vi "3_AdvancedDemo_MHT3.vi"() -> ()   [LabVIEW 2010]
uses:
  Types/MH_UIThread_Cmds.ctl
  _lib/PQ/MultiHarp/MH_InitInfo.ctl
  Types/MH_UIThread_Data.ctl
  Types/MH_InputChannel.ctl
  _lib/PQ/MultiHarp/MH_RefSource.ctl
  _lib/PQ/MultiHarp/mhlib_x86_x64_UIThread.llb/MH_DllPath_global.vi
  <vilib>/Utility/error.llb/DialogType.ctl
  Types/MH_DataProcThread_QCmds.ctl
  Types/MH_DataProcThread_QData.ctl
  Types/MH_VisThread_QCmds.ctl
  Types/MH_VisThread_QData.ctl
  Types/MH_VisThread_Data.ctl
  _lib/PQ/MultiHarp/MH_LibVersion_global.vi
  _lib/PQ/MultiHarp/MH_MeasMode.ctl
panel:
  in  "Settings":bool=TRUE
  in  "Run continuously":bool caption="Conti."
  in  "Start":bool
  in  "Scale":bool
  out "CountRates":i32[](graph)
  in  "HistoAcqTime":dbl=1.0 caption="Int.Time    s" min=0.1 max=360000.0 step=0.1
  in  "AcqTime":i32=360000000 caption="T3Acq.   ms" min=1 max=360000 step=1
  in  "Binning":i32(ring) caption="Resol.      ps" items=["80", "160", "320", "640", "1280", "2560", "5120", "10240", "20480", "40960", "81920", "163840", "327680", "655360", "1310720", "2621440", "5242880", "10485760", "20971520", "41943040", "83886080", "167772160", "335544320", "671088640", "1342177280", "2684354560"]
  in  "HistoOffset":i32 caption="Offset      ns" min=0 max=100000000 step=1
  out "DeltaT":dbl=3.2767475720388473 caption="Resol.     ms" format="%.2f"
  in  "BitShift":i32=15 min=0 max=32 step=1
  in  "OvlLevel":i32=65536 caption="Ovl.Level" min=1024 max=65536 step=1024
  in  "StopOvl.":bool=TRUE
  out "TTraceGraph":T1(graph)={0.0, "Resolution"=0.0032767475720388473, "Histogram"=[]}
  out "HistoGraph":cluster{dbl, "Resol":dbl, "Histos":u32[][]}(graph)={0.0, "Resol"=0.08, "Histos"=[]}
  in  "SyncEdge":i32(ring) caption="Edge" items=["falling", "rising"]
  in  "SyncDivider":i32(ring)=3 caption="Divider" items=["1", "2", "4", "8", "16"]
  in  "SyncOffset":i32 caption="Offset      ps" min=-99999 max=99999 step=1
  in  "SyncLevel":i32=-50 caption="Level      mV" min=-1200 max=1200 step=1
  in  "Channels":T2[](array[typedef])=[{"Name"="Inp.Chan 1", "Enable"=TRUE, "Offset"=0, "Level"=-50, "Edge"=0}, {"Name"="Inp.Chan 2", "Enable"=TRUE, "Offset"=0, "Level"=-50, "Edge"=0}, {"Name"="Inp.Chan 3", "Enable"=TRUE, "Offset"=0, "Level"=-50, "Edge"=0}, {"Name"="Inp.Chan 4", "Enable"=TRUE, "Offset"=0, "Level"=-50, "Edge"=0}, {"Name"="Inp.Chan 5", "Enable"=TRUE, "Offset"=0, "Level"=-50, "Edge"=0}, {"Name"="Inp.Chan 6", "Enable"=TRUE, "Offset"=0, "Level"=-50, "Edge"=0}, {"Name"="Inp.Chan 7", "Enable"=TRUE, "Offset"=0, "Level"=-50, "Edge"=0}, {"Name"="Inp.Chan 8", "Enable"=TRUE, "Offset"=0, "Level"=-50, "Edge"=0}] {"Edge" items=["falling", "rising"]; "Offset" min=-99999 max=99999 step=80; "Level" min=-1200 max=1200 step=1}
  out "SyncRate":string="Sync Rate: 10000160 cps\n"
  out "OverRun":bool caption="Overrun:"
  out "Status":string="Elements in Q: 0"
  # "Histogram"
  # "Time Trace"
  # "Sync"
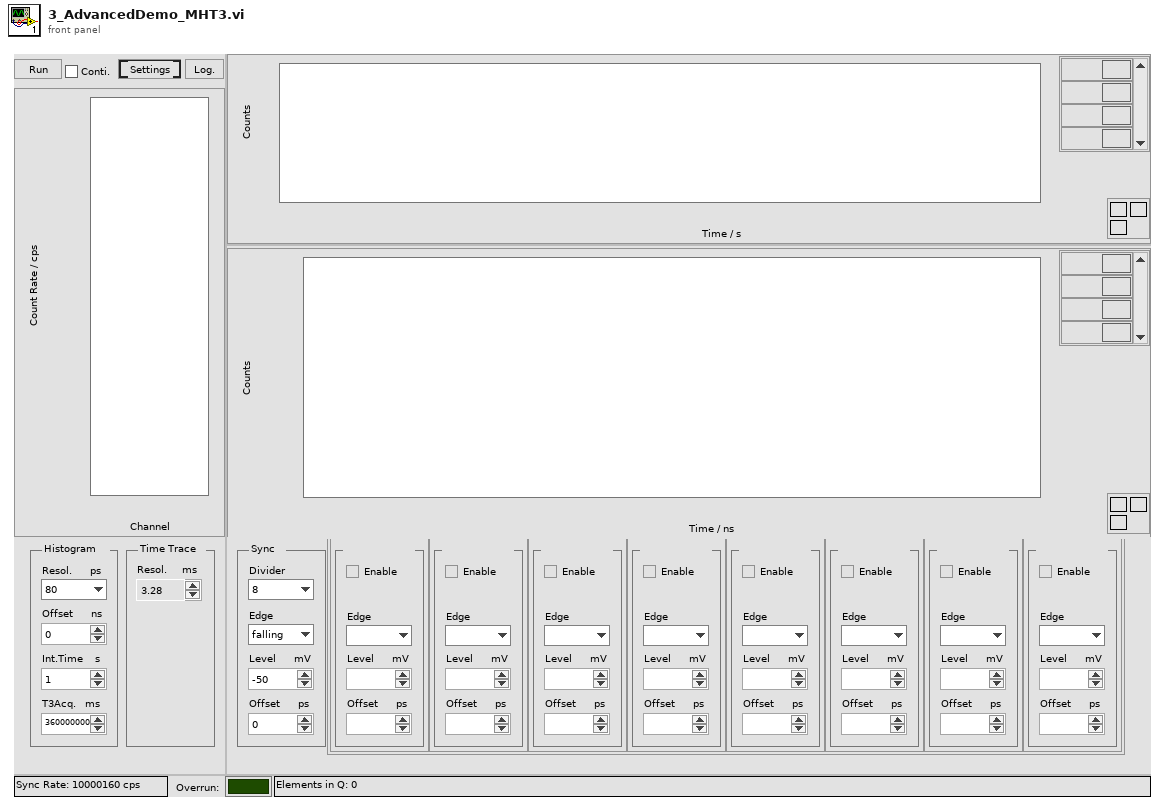
[diagram p1: front panel]
types:
  T1 = cluster{dbl, "Resolution":dbl, "Histogram":u32[][]}
  T2 = typedef "MH_InputChannel.ctl" = cluster{"Name":string, "Enable":bool, "Offset":i32, "Level":i32, "Edge":i32}
  T3 = typedef "MH_DataProcThread_QCmds.ctl" = enum16{"Exit", "Proc", "Init", "SetShift", "SetNumChannels", "SetHistAcqTime"}
  T4 = typedef "MH_VisThread_Data.ctl" = cluster{"Resol":dbl, "DeltaT":dbl, "NumChannels":i32}
  T5 = typedef "MH_VisThread_QData.ctl" = cluster{"Histos":u32[][], "Cmd":T6, "TimeTrace":u32[][], "Bin":i32, "Total bin":u64, "Status":string, "Resol":dbl, "DeltaT":dbl, "nChannels":i32}
  T6 = typedef "MH_VisThread_QCmds.ctl" = enum16{"_none_", "Resol", "nChannels", "DeltaT", "Histo", "TTrace", "Status"}
  T7 = typedef "MH_DataProcThread_QData.ctl" = cluster{"Cmd":T3, "nActual":i32, "Buffer":u32[], "TickCount":u32, "Param":i32}
  T8 = typedef "MH_UIThread_Data.ctl" = cluster{"Init Info":T9, "DevIdx":i32, "SyncDivider":i32, "SyncOffset":i32, "SyncLevel":i32, "Channels":T2[], "CurrentChannels":i32[], "AcqTime":i32, "Binning":i32, "HistoOffset":i32, "HistoLen":i32, "StopOvl.":bool, "OvlLevel":u32, "SyncEdge":i32, "StartMeas":bool, "HistoLength":i32, "Resolution":dbl, "Run cont.":bool, "Status":string, "SyncRate":i32, "BitShift":i32, "HistoAcqTime":dbl}
  T9 = typedef "MH_InitInfo.ctl" = cluster{"Library Version":string, "Serial No.":string, "Model":string, "Partnum":string, "Version":string, "features":i32, "nchannels":i32, "Base Resolution":dbl, "Bin Steps":i32}
  T10 = typedef "MH_UIThread_Cmds.ctl" = enum16{"Idle", "Init", "SetInpChanEnable", "SetInpChanOffset", "SetInpChanTrg", "SetSyncDivider", "SetSyncTrg", "SetSyncOffset", "SetBinning", "SetHistoOffset", "SetHistoLen", "SetStopOvl", "SetBitShift", "SetHistoAcqTime", "GetRates", "GetAllRates", "StartMeas", "StopMeas", "AbortMeas", "GetResolution", "GetHistos", "GetAllHistos", "ReadFiFo", "WriteStatus", "Resize", "EnableControls", "DisableControls", "Error", "Exit"}
  T11 = enum8{"Enabled", "Disabled", "Disabled and Grayed Out"}
  T12 = typedef "MH_MeasMode.ctl" = i32
  T13 = typedef "MH_RefSource.ctl" = enum16{"INTERNAL", "EXTERNAL_10MHZ", "WR_MASTER_GENERIC", "WR_SLAVE_GENERIC", "WR_GRANDM_GENERIC", "EXTN_GPS_PPS", "EXTN_GPS_PPS_UART", "WR_MASTER_MHARP", "WR_SLAVE_MHARP", "WR_GRANDM_MHARP"}
  T14 = typedef "DialogType.ctl" = u16
  T15 = cluster{"T0":dbl, "dt":dbl, "TimeTrace_out":u32[][]}
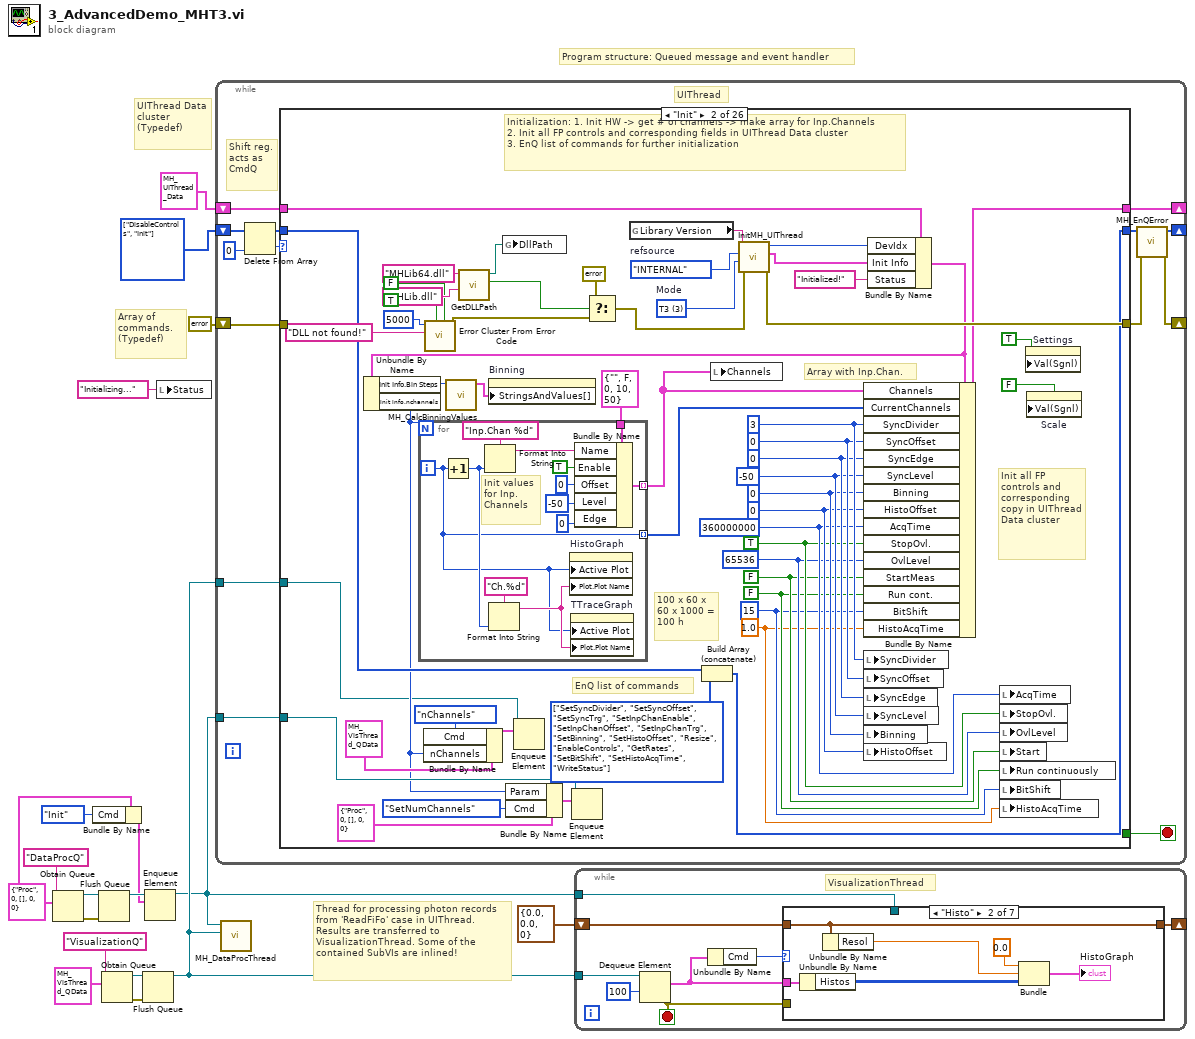
[diagram p0: block diagram]
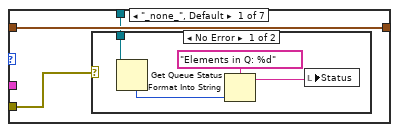
[diagram p2: hidden frame]
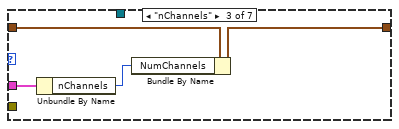
[diagram p4: hidden frame]
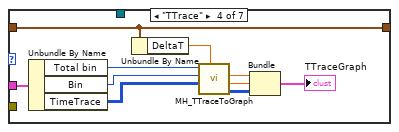
[diagram p5: hidden frame]
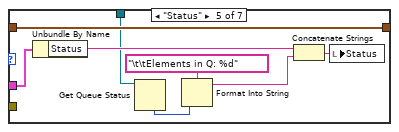
[diagram p6: hidden frame]
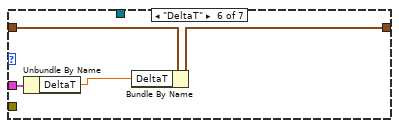
[diagram p7: hidden frame]
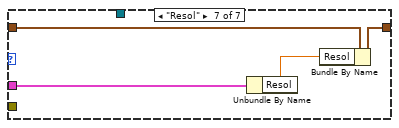
[diagram p8: hidden frame]
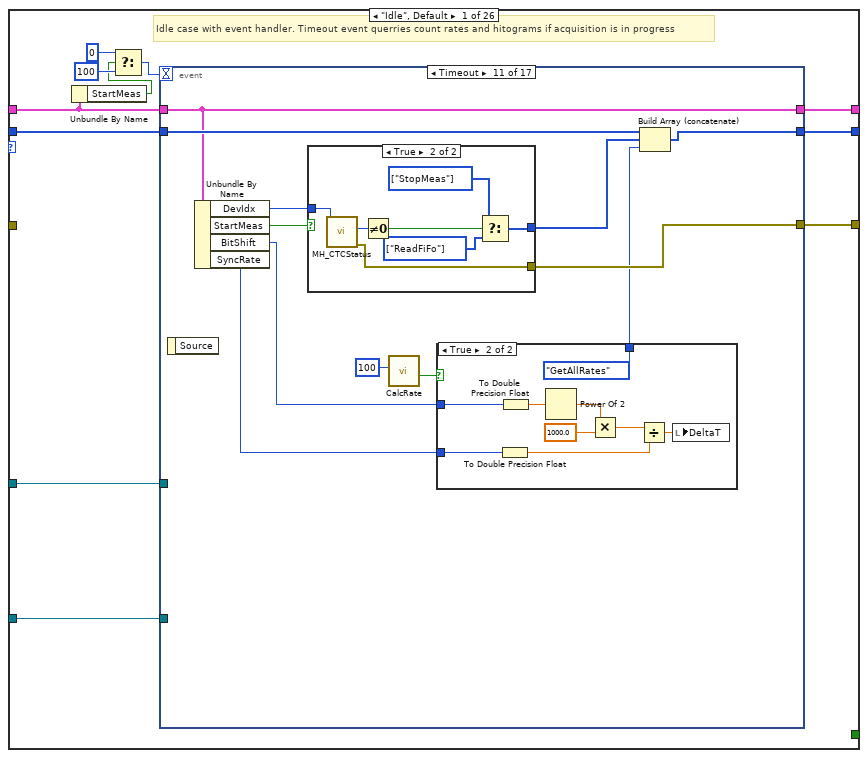
[diagram p9: hidden frame]
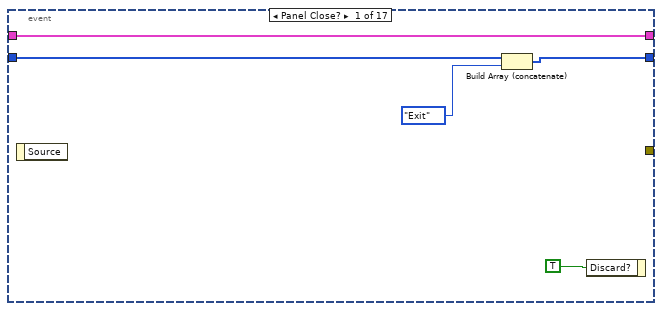
[diagram p10: hidden frame]
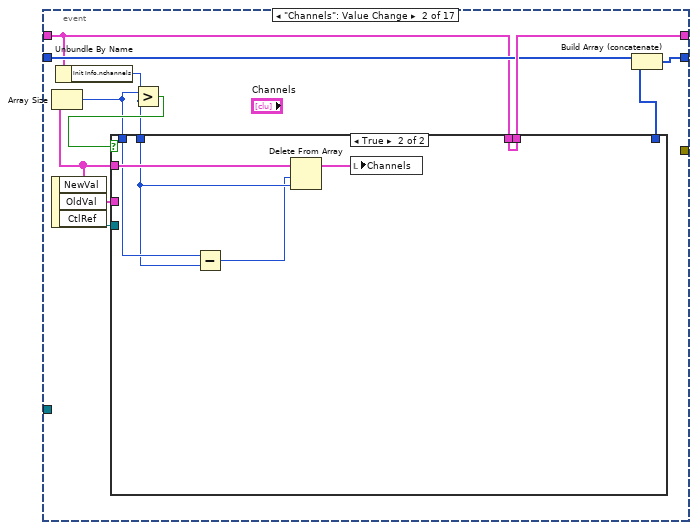
[diagram p11: hidden frame]
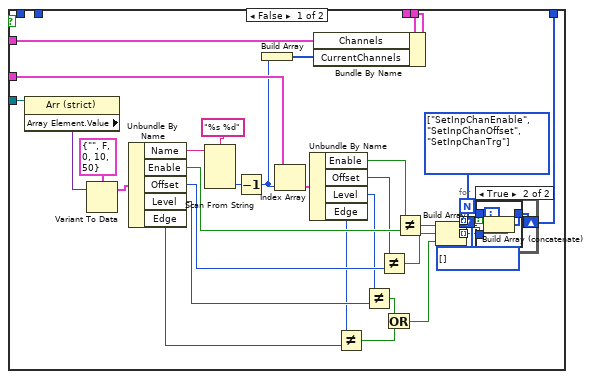
[diagram p12: hidden frame]
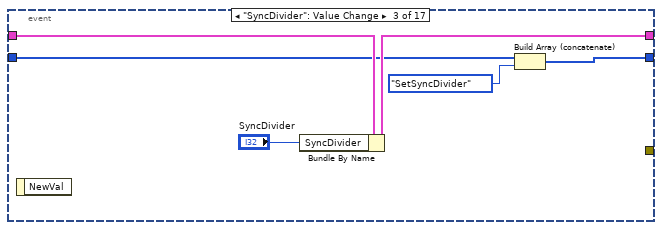
[diagram p14: hidden frame]
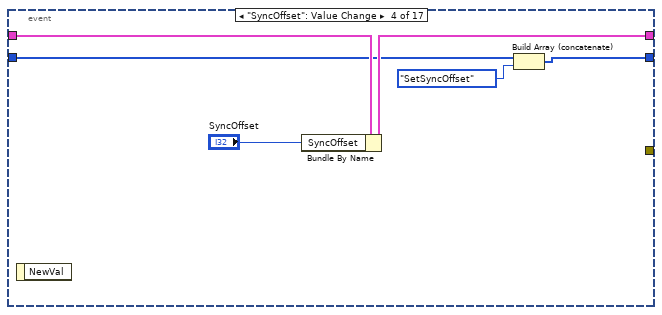
[diagram p15: hidden frame]
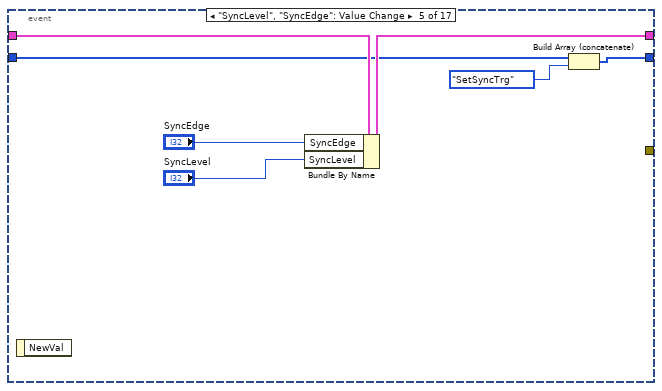
[diagram p16: hidden frame]
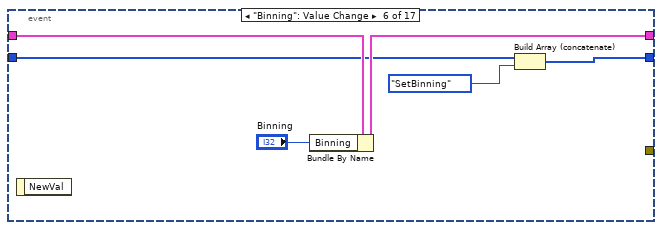
[diagram p17: hidden frame]
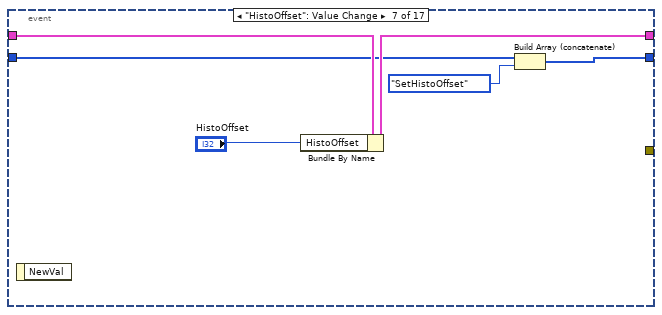
[diagram p18: hidden frame]
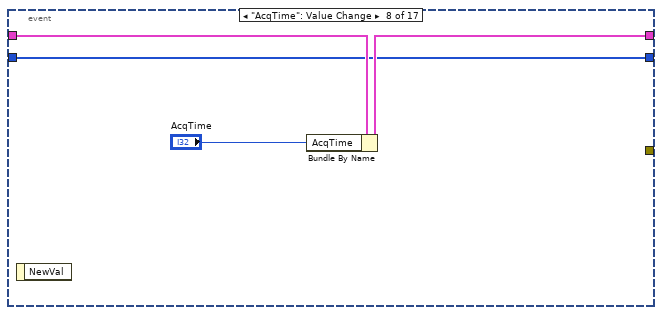
[diagram p19: hidden frame]
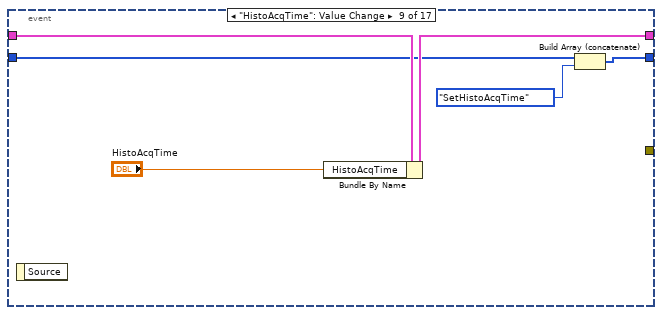
[diagram p20: hidden frame]
diagram:
  w4 = T7 {"Cmd"=enum."Proc", "nActual"=0, "Buffer"=[], "TickCount"=0, "Param"=0} ("MH_DataProcThread_QData")
  w17 = T10[] [enum."DisableControls", enum."Init"] items=["Idle", "Init", "SetInpChanEnable", "SetInpChanOffset", "SetInpChanTrg", "SetSyncDivider", "SetSyncTrg", "SetSyncOffset", "SetBinning", "SetHistoOffset", "SetHistoLen", "SetStopOvl", "SetBitShift", "SetHistoAcqTime", "GetRates", "GetAllRates", "StartMeas", "StopMeas", "AbortMeas", "GetResolution", "GetHistos", "GetAllHistos", "ReadFiFo", "WriteStatus", "Resize", "EnableControls", "DisableControls", "Error", "Exit"]
  # "Thread for processing photon records from 'ReadFiFo' case in UIThread. Results are transferred to VisualizationThread. Some of the contained SubVIs are inlined!"
  # "Array of commands.\n(Typedef)"
  # "Program structure: Queued message and event handler"
  # "UIThread Data cluster\n(Typedef)"
  n1 = Obtain Queue(name (unnamed)="DataProcQ", element data type=w4) -> (queue out=w14:refnum<queue>, error out=w13:errorcluster)  [unwired: 3 in, 1 out]
  n2 = Bundle By Name(cluster=w4, "Cmd"=MH_DataProcThread_QCmds."Init") -> (w2:T7)
  n3 = Flush Queue(queue=w14, error in (no error)=w13) -> (queue out=w5:refnum<queue>)  [unwired: 2 out]
  n4 = Obtain Queue(name (unnamed)="VisualizationQ", element data type=T5 {"Histos"=[], "Cmd"=enum."_none_", "TimeTrace"=[], "Bin"=0, "Total bin"=0, "Status"="", "Resol"=0.0, "DeltaT"=0.0, "nChannels"=0} ("MH_GUIThread_QData")) -> (queue out=w12:refnum<queue>, error out=w11:errorcluster)  [unwired: 3 in, 1 out]
  n5 = Flush Queue(queue=w12, error in (no error)=w11) -> (queue out=w7:refnum<queue>)  [unwired: 2 out]
  n6 = Enqueue Element(queue=w5, element=w2) -> (queue out=w1:refnum<queue>)  [unwired: 2 in, 2 out]
  n7 = local write "Status"("Initializing..." ("Status")) -> ()
  n8 = while {
    shift-right: [w21] -> _
    shift-left: w17 -> [w28]
    shift-right: [w31] -> _
    shift-left: T8 {"Init Info"={"Library Version"="", "Serial No."="", "Model"="", "Partnum"="", "Version"="", "features"=0, "nchannels"=0, "Base Resolution"=0.0, "Bin Steps"=0}, "DevIdx"=0, "SyncDivider"=1, "SyncOffset"=0, "SyncLevel"=50, "Channels"=[], "CurrentChannels"=[], "AcqTime"=1, "Binning"=1, "HistoOffset"=1, "HistoLen"=1024, "StopOvl."=FALSE, "OvlLevel"=1024, "SyncEdge"=10, "StartMeas"=FALSE, "HistoLength"=0, "Resolution"=0.0, "Run cont."=FALSE, "Status"="", "SyncRate"=0, "BitShift"=0, "HistoAcqTime"=0.0} -> [w30]
    shift-right: [w23] -> _
    shift-left: errorcluster {"status"=FALSE, "code"=0, "source"=""} ("error IO") -> [w29]
    tunnel: w1 -> [w20]
    tunnel: w7 -> [w19]
    stop <- w32 stop-if-true
    # "Shift reg.\nacts as\nCmdQ"
    # "UIThread"
    n9 = Delete From Array(array=w28, index=0) -> (deleted portion=w26:T10, array with subset deleted=w25:T10[])  [unwired: 1 in]
    n10 = case shown="\"Init\"" w26 {
      tunnel: [w43 w283 w307 w321 w335 w352 w361 w363 w370 w378 w385 w405 w417 w427 w439 w459 w465 w478 w495 w496 w522 w535 w542 w554 w560 w566] -> w22
      tunnel: [_ _ _ _ _ _ _ _ _ _ _ _ _ _ _ _ _ _ _ _ _ _ _ _ _ TRUE] -> w32
      tunnel: [w42 w264 w310 w324 w338 w354 w362 w367 w374 w379 w386 w390 w407 w421 w431 w463 w468 w480 w491 w506 w521 w523 w541 w553 w561 w569] -> w31
      tunnel: w30 -> [w39 w269 w310 w324 w338 w354 w362 w367 w374 w379 w386 w390 w407 w421 w432 w463 w469 w481 w492 w506 w521 w523 w541 w553 w561 w569]
      tunnel: [w40 w288 w308 w322 w336 w350 w360 w366 w373 w377 w384 _ _ w420 w438 w462 w471 w483 w493 w501 _ _ _ _ _ w567] -> w24
      tunnel: w29 -> [_ _ _ _ _ _ _ _ _ _ _ _ _ _ _ _ _ _ _ _ _ _ _ _ w562 _]
      tunnel: w25 -> [w41 w285 w307 w321 w335 w352 w361 w363 w369 w378 w385 w405 w417 w427 w439 w460 w466 w478 w495 w497 w522 w535 w542 w554 _ w566]
      tunnel: w20 -> [w34 w262 _ _ _ _ _ _ _ _ _ w391 w408 _ _ w456 _ _ _ w498 _ _ _ _ _ w565]
      tunnel: w19 -> [w33 w254 _ _ _ _ _ _ _ _ _ w392 _ _ _ _ _ _ w488 _ _ _ _ _ _ w564]
      frame "Idle", Default {
        # "Idle case with event handler. Timeout event querries count rates and hitograms if acquisition is in progress"
        n11 = Unbundle By Name(w39) -> ("StartMeas"=w37:bool)
        n12 = Select(t=0, s=w37, f=100) -> (s? t:f=w36:i32)
        n13 = event shown="[10] Timeout" {
          selector: _ -> [_ _ _ _ _ _ _ _ _ _ _ _ _ _ _ _ _]
          dyn-events: _ -> [_ _ _ _ _ _ _ _ _ _ _ _ _ _ _ _ _]
          timeout: w36 -> [_ _ _ _ _ _ _ _ _ _ _ _ _ _ _ _ _]
          tunnel: [w44 w54 w105 w111 w118 w125 w131 w136 w141 w148 w163 w181 w193 w211 w217 w225 w235] -> w43
          tunnel: [w47 w57 w109 w115 w122 w128 w134 w138 w144 w151 w162 w185 w192 w209 w216 w224 w238] -> w42
          tunnel: w39 -> [w47 w53 w110 w116 w123 w129 w135 w139 w145 w152 w162 w186 w190 w210 w216 w224 w238]
          tunnel: w41 -> [w46 w56 w107 w113 w120 w127 w133 w136 w142 w150 w164 w182 w194 w211 w217 w225 w236]
          tunnel: [_ _ _ _ _ _ _ _ _ _ w158 _ _ _ _ _ _] -> w40
          tunnel: w34 -> [_ _ _ _ _ _ _ _ _ _ _ _ _ _ _ _ _]
          tunnel: w33 -> [_ _ _ _ _ _ _ _ _ _ _ _ _ _ _ _ _]
          event Panel Close? {
            n14 = event-data() -> ()  [unwired: 1 in, 1 out]
            n15 = Build Array (concatenate)(w46, MH_UIThread_Cmds."Exit") -> (w44:T10[])
            n16 = event-data("Discard?"=TRUE) -> ()  [unwired: 1 in, 1 out]
          }
          event "Channels": Value Change {
            n17 = event-data() -> ("NewVal"=w52:T2[], "OldVal"=w58:T2[], "CtlRef"=w59:refnum<vi>)  [unwired: 1 in]
            n18 = Array Size(array=w52) -> (size(s)=w49:i32)
            n19 = Unbundle By Name(w53) -> ("Init Info.nchannels"=w50:i32)
            n20 = Greater?(x=w49, y=w50) -> (0:w51:bool)
            n21 = case shown="True" w51 {
              tunnel: w59 -> [w90 _]
              tunnel: w58 -> [w84 _]
              tunnel: [w67 w104] -> w57
              tunnel: [w65 _] -> w55
              tunnel: w53 -> [w62 w104]
              tunnel: w52 -> [w61 w103]
              tunnel: w50 -> [_ w101]
              tunnel: w49 -> [_ w102]
              frame False {
                w60 = T10[] [] items=["Idle", "Init", "SetInpChanEnable", "SetInpChanOffset", "SetInpChanTrg", "SetSyncDivider", "SetSyncTrg", "SetSyncOffset", "SetBinning", "SetHistoOffset", "SetHistoLen", "SetStopOvl", "SetBitShift", "SetHistoAcqTime", "GetRates", "GetAllRates", "StartMeas", "StopMeas", "AbortMeas", "GetResolution", "GetHistos", "GetAllHistos", "ReadFiFo", "WriteStatus", "Resize", "EnableControls", "DisableControls", "Error", "Exit"] ("Array")
                w68 = T10[] [enum."SetInpChanEnable", enum."SetInpChanOffset", enum."SetInpChanTrg"] items=["Idle", "Init", "SetInpChanEnable", "SetInpChanOffset", "SetInpChanTrg", "SetSyncDivider", "SetSyncTrg", "SetSyncOffset", "SetBinning", "SetHistoOffset", "SetHistoLen", "SetStopOvl", "SetBitShift", "SetHistoAcqTime", "GetRates", "GetAllRates", "StartMeas", "StopMeas", "AbortMeas", "GetResolution", "GetHistos", "GetAllHistos", "ReadFiFo", "WriteStatus", "Resize", "EnableControls", "DisableControls", "Error", "Exit"]
                n22 = property class="Arr (strict)"(reference=w90) -> ("Array Element.Value"=w89:variant)  [unwired: 1 in, 2 out]
                n23 = Variant To Data(Variant=w89, type=T2 {"Name"="", "Enable"=FALSE, "Offset"=0, "Level"=10, "Edge"=50} ("Channel")) -> (data=w66:cluster{})  [unwired: 1 in, 1 out]
                n24 = Unbundle By Name(w66) -> ("Name"=w87:string, "Enable"=w81:bool, "Offset"=w79:i32, "Level"=w77:i32, "Edge"=w75:i32)
                n25 = Scan From String(format string="%s %d", input string=w87) -> (output 2=w85:i32)  [unwired: 5 in, 3 out]
                n26 = Decrement(x=w85) -> (x-1=w64:i32)
                n27 = Build Array(w64) -> (w63:i32[])
                n28 = Index Array(array=w84, index=w64) -> (element=w83:T2)
                n29 = Unbundle By Name(w83) -> ("Enable"=w82:bool, "Offset"=w80:i32, "Level"=w78:i32, "Edge"=w76:i32)
                n30 = Bundle By Name(cluster=w62, "Channels"=w61, "CurrentChannels"=w63) -> (w67:T8)
                n31 = Not Equal?(x=w76, y=w75) -> (x != y?=w70:bool)
                n32 = Not Equal?(x=w78, y=w77) -> (x != y?=w71:bool)
                n33 = Not Equal?(x=w80, y=w79) -> (x != y?=w73:bool)
                n34 = Or(x=w71, y=w70) -> (x .or. y?=w69:bool)
                n35 = Not Equal?(x=w82, y=w81) -> (x != y?=w74:bool)
                n36 = Build Array(w74, w73, w69) -> (w72:bool[])
                n37 = for {
                  tunnel: w72 -> [w93] mode=indexing
                  tunnel: w68 -> [w94] mode=indexing
                  shift-right: [w91] -> w65
                  shift-left: w60 -> [w92]
                  n38 = case shown="True" w93 {
                    tunnel: w92 -> [w95 w97]
                    tunnel: w94 -> [_ w96]
                    tunnel: [w95 w98] -> w91
                    frame False {
                    }
                    frame True {
                      n39 = Build Array (concatenate)(w97, w96) -> (w98:T10[])
                    }
                  }
                }
              }
              frame True {
                n40 = Subtract(x=w102, y=w101) -> (x-y=w100:i32)
                n41 = Delete From Array(array=w103, length=w100, index=w101) -> (array with subset deleted=w99:T2[])  [unwired: 1 out]
                n42 = local write "Channels"(w99) -> ()
              }
            }
            n43 = Build Array (concatenate)(w56, w55) -> (w54:T10[])
          }
          event "SyncDivider": Value Change {
            n44 = event-data() -> ()  [unwired: 1 in, 1 out]
            n45 = Bundle By Name(cluster=w110, "SyncDivider"="SyncDivider") -> (w109:T8)
            n46 = Build Array (concatenate)(w107, MH_UIThread_Cmds."SetSyncDivider") -> (w105:T10[])
          }
          event "SyncOffset": Value Change {
            n47 = event-data() -> ()  [unwired: 1 in, 1 out]
            n48 = Bundle By Name(cluster=w116, "SyncOffset"="SyncOffset") -> (w115:T8)
            n49 = Build Array (concatenate)(w113, MH_UIThread_Cmds."SetSyncOffset") -> (w111:T10[])
          }
          event "SyncLevel", "SyncEdge": Value Change {
            n50 = event-data() -> ()  [unwired: 1 in, 1 out]
            n51 = Bundle By Name(cluster=w123, "SyncEdge"="SyncEdge", "SyncLevel"="SyncLevel") -> (w122:T8)
            n52 = Build Array (concatenate)(w120, MH_UIThread_Cmds."SetSyncTrg") -> (w118:T10[])
          }
          event "Binning": Value Change {
            n53 = event-data() -> ()  [unwired: 1 in, 1 out]
            n54 = Bundle By Name(cluster=w129, "Binning"="Binning") -> (w128:T8)
            n55 = Build Array (concatenate)(w127, MH_UIThread_Cmds."SetBinning") -> (w125:T10[])
          }
          event "HistoOffset": Value Change {
            n56 = event-data() -> ()  [unwired: 1 in, 1 out]
            n57 = Bundle By Name(cluster=w135, "HistoOffset"="HistoOffset") -> (w134:T8)
            n58 = Build Array (concatenate)(w133, MH_UIThread_Cmds."SetHistoOffset") -> (w131:T10[])
          }
          event "AcqTime": Value Change {
            n59 = event-data() -> ()  [unwired: 1 in, 1 out]
            n60 = Bundle By Name(cluster=w139, "AcqTime"="AcqTime") -> (w138:T8)
          }
          event "HistoAcqTime": Value Change {
            n61 = event-data() -> ()  [unwired: 1 in, 1 out]
            n62 = Bundle By Name(cluster=w145, "HistoAcqTime"="HistoAcqTime") -> (w144:T8)
            n63 = Build Array (concatenate)(w142, MH_UIThread_Cmds."SetHistoAcqTime") -> (w141:T10[])
          }
          event "OvlLevel", "StopOvl.": Value Change {
            n64 = event-data() -> ()  [unwired: 1 in, 1 out]
            n65 = Bundle By Name(cluster=w152, "StopOvl."="StopOvl.", "OvlLevel"="OvlLevel") -> (w151:T8)
            n66 = Build Array (concatenate)(w150, MH_UIThread_Cmds."SetStopOvl") -> (w148:T10[])
          }
          event Timeout {
            n67 = event-data() -> ()  [unwired: 1 in, 1 out]
            n68 = Unbundle By Name(w162) -> ("DevIdx"=w160:i32, "StartMeas"=w161:bool, "BitShift"=w157:i32, "SyncRate"=w156:i32)
            n69 = case shown="True" w161 {
              tunnel: w160 -> [_ w180]
              tunnel: [_ w178] -> w159
              tunnel: [_ w175] -> w158
              frame False {
              }
              frame True {
                w176 = T10[] [enum."ReadFiFo"] items=["Idle", "Init", "SetInpChanEnable", "SetInpChanOffset", "SetInpChanTrg", "SetSyncDivider", "SetSyncTrg", "SetSyncOffset", "SetBinning", "SetHistoOffset", "SetHistoLen", "SetStopOvl", "SetBitShift", "SetHistoAcqTime", "GetRates", "GetAllRates", "StartMeas", "StopMeas", "AbortMeas", "GetResolution", "GetHistos", "GetAllHistos", "ReadFiFo", "WriteStatus", "Resize", "EnableControls", "DisableControls", "Error", "Exit"]
                w177 = T10[] [enum."StopMeas"] items=["Idle", "Init", "SetInpChanEnable", "SetInpChanOffset", "SetInpChanTrg", "SetSyncDivider", "SetSyncTrg", "SetSyncOffset", "SetBinning", "SetHistoOffset", "SetHistoLen", "SetStopOvl", "SetBitShift", "SetHistoAcqTime", "GetRates", "GetAllRates", "StartMeas", "StopMeas", "AbortMeas", "GetResolution", "GetHistos", "GetAllHistos", "ReadFiFo", "WriteStatus", "Resize", "EnableControls", "DisableControls", "Error", "Exit"]
                n70 = call "MH_CTCStatus.vi"("devidx"=w180) -> ("error out"=w175:errorcluster, "ctcstatus"=w179:i32)  [unwired: 8 in, 1 out]
                n71 = Not Equal To 0?(x=w179) -> (x != 0?=w174:bool)
                n72 = Select(t=w177, s=w174, f=w176) -> (s? t:f=w178:T10[])
              }
            }
            n73 = call "CalcRate.vi"("Refresh(ms)"=u32 100) -> ("updated?"=w154:bool)  [unwired: 8 in, 2 out]
            n74 = case shown="True" w154 {
              tunnel: w157 -> [_ w167]
              tunnel: w156 -> [_ w166]
              tunnel: [_ MH_UIThread_Cmds."GetAllRates"] -> w155
              frame False {
              }
              frame True {
                n75 = To Double Precision Float(number=w166) -> (double precision float=w171:dbl)
                n76 = To Double Precision Float(number=w167) -> (double precision float=w172:dbl)
                n77 = Power Of 2(x=w172) -> (2^x=w170:dbl)
                n78 = Multiply(x=w170, y=1000.0) -> (x*y=w169:dbl)
                n79 = Divide(x=w169, y=w171) -> (x/y=w173:dbl)
                n80 = local write "DeltaT"(w173) -> ()
              }
            }
            n81 = Build Array (concatenate)(w164, w159, w155) -> (w163:T10[])
          }
          event "BitShift": Value Change {
            n82 = event-data() -> ()  [unwired: 1 in, 1 out]
            n83 = Bundle By Name(cluster=w186, "BitShift"="BitShift") -> (w185:T8)
            n84 = Build Array (concatenate)(w182, MH_UIThread_Cmds."SetBitShift") -> (w181:T10[])
          }
          event "Start": Value Change {
            n85 = event-data() -> ()  [unwired: 1 in, 1 out]
            n86 = Unbundle By Name(w190) -> ("SyncRate"=w189:i32)
            n87 = Greater Or Equal?(x=w189, y=10) -> (x >= y?=w187:bool)
            n88 = case shown="True" w187 {
              selector: w187 -> [w196 _]
              tunnel: w194 -> [w198 w207]
              tunnel: [w198 w205] -> w193
              tunnel: [w197 w204] -> w192
              tunnel: "Start" -> [_ w203]
              tunnel: w190 -> [w197 w199]
              frame False {
                n89 = local write "Start"(w196) -> ()
                n90 = One Button Dialog(message="SyncRate too low!!!" ("Status")) -> ()  [unwired: 1 in, 1 out]
              }
              frame True {
                w202 = T10[] [enum."SetBitShift", enum."SetHistoAcqTime", enum."StartMeas"] items=["Idle", "Init", "SetInpChanEnable", "SetInpChanOffset", "SetInpChanTrg", "SetSyncDivider", "SetSyncTrg", "SetSyncOffset", "SetBinning", "SetHistoOffset", "SetHistoLen", "SetStopOvl", "SetBitShift", "SetHistoAcqTime", "GetRates", "GetAllRates", "StartMeas", "StopMeas", "AbortMeas", "GetResolution", "GetHistos", "GetAllHistos", "ReadFiFo", "WriteStatus", "Resize", "EnableControls", "DisableControls", "Error", "Exit"]
                n91 = Bundle By Name(cluster=w199, "StartMeas"=w203) -> (w204:T8)
                n92 = Build Array(MH_UIThread_Cmds."AbortMeas") -> (w200:T10[])
                n93 = Select(t=w202, s=w203, f=w200) -> (s? t:f=w206:T10[])
                n94 = Build Array (concatenate)(w207, w206) -> (w205:T10[])
              }
            }
          }
          event "Run continuously": Value Change {
            n95 = event-data() -> ()  [unwired: 1 in, 1 out]
            n96 = Bundle By Name(cluster=w210, "Run cont."="Run continuously") -> (w209:T8)
          }
          event "Scale": Value Change {
            n97 = event-data() -> ()  [unwired: 1 in, 1 out]
            n98 = Select(t=u8 0 ("Y Scale.Mapping Mode"), s="Scale", f=u8 1 ("Y Scale.Mapping Mode")) -> (s? t:f=w212:u8)
            n99 = property on="HistoGraph" class="WFGraph (strict)"("YScale.Mapping Mode"=w212) -> ()  [unwired: 2 in, 2 out]
          }
          event "Settings": Value Change {
            n100 = event-data() -> ()  [unwired: 1 in, 1 out]
            n101 = property on="Splitter" class="Splitter"() -> ("Position"=w223:i32)  [unwired: 2 in, 2 out]
            n102 = Select(t=237 ("PosT"), s="Settings", f=0 ("PosF")) -> (s? t:f=w220:i32)
            n103 = Subtract(x=w223, y=w220) -> (x-y=w219:i32)
            n104 = while {
              shift-right: [w234] -> _
              shift-left: w219 -> [w227]
              i -> [w233]
              stop <- w230 stop-if-true
              n105 = property on="Splitter 4" class="Splitter"("Position"=w227) -> (error out=w226:errorcluster)  [unwired: 2 in, 1 out]
              n106 = Greater Or Equal?(x=w233, y=10) -> (x >= y?=w231:bool)
              n107 = Decrement(x=w227) -> (x-1=w234:i32)
              n108 = Unbundle(w226) -> ("status"=w229:bool)  [unwired: 2 out]
              n109 = Not(x=w229) -> (.not. x?=w228:bool)
              n110 = Or(x=w228, y=w231) -> (x .or. y?=w230:bool)
            }
          }
          event Panel Resize {
            n111 = event-data() -> ()  [unwired: 1 in, 1 out]
            n112 = Build Array (concatenate)(w236, MH_UIThread_Cmds."Resize") -> (w235:T10[])
          }
        }
      }
      frame "Init" {
        w243 = T12 3 items=["HIST"=0, "T2"=2, "T3"=3]  # Mode
        w245 = MH_RefSource."INTERNAL"  # refsource
        w252 = 1.0 ("HistoAcqTime")
        w253 = 15 ("Value (Signaling)")
        w271 = FALSE ("Run cont.")
        w273 = FALSE ("StartMeas")
        w274 = 65536 ("OvlLevel")
        w275 = TRUE ("StopOvl.")
        w276 = 360000000 ("AcqTime")
        w277 = 0 ("HistoOffset")
        w278 = 0 ("Binning")
        w279 = -50 ("SyncLevel")
        w280 = 0 ("SyncZeroX")
        w281 = 0 ("SyncOffset")
        w282 = 3 ("SyncDivider")
        w284 = T10[] [enum."SetSyncDivider", enum."SetSyncOffset", enum."SetSyncTrg", enum."SetInpChanEnable", enum."SetInpChanOffset", enum."SetInpChanTrg", enum."SetBinning", enum."SetHistoOffset", enum."Resize", enum."EnableControls", enum."GetRates", enum."SetBitShift", enum."SetHistoAcqTime", enum."WriteStatus"] items=["Idle", "Init", "SetInpChanEnable", "SetInpChanOffset", "SetInpChanTrg", "SetSyncDivider", "SetSyncTrg", "SetSyncOffset", "SetBinning", "SetHistoOffset", "SetHistoLen", "SetStopOvl", "SetBitShift", "SetHistoAcqTime", "GetRates", "GetAllRates", "StartMeas", "StopMeas", "AbortMeas", "GetResolution", "GetHistos", "GetAllHistos", "ReadFiFo", "WriteStatus", "Resize", "EnableControls", "DisableControls", "Error", "Exit"]
        # "100 x 60 x 60 x 1000 = 100 h"
        # "Init all FP controls and corresponding copy in UIThread Data cluster"
        # "EnQ list of commands"
        # "Array with Inp.Chan."
        # "Initialization: 1. Init HW -> get # of channels -> make array for Inp.Channels\n2. Init all FP controls and corresponding fields in UIThread Data cluster\n3. EnQ list of commands for further initialization"
        n113 = call <vilib>:"Error Cluster From Error Code.vi"("is warning? (False)"=FALSE, "show call chain? (False)"=TRUE, "error message (\"\")"="DLL not found!" ("error message (\"\")"), "error code (0)"=5000) -> ("error out"=w246:errorcluster)  [unwired: 5 in]
        n114 = call "GetDLLPath.vi"("DllName_32bit"="MHLib.dll" ("name or relative path"), "DllName_64bit"="MHLib64.dll" ("name or relative path")) -> ("file exists?"=w248:bool, "DLLPath"=w249:path)  [unwired: 8 in]
        n115 = global write "MH_DllPath_global.vi" "DllPath"(w249) -> ()
        n116 = Select(t=errorcluster {"status"=FALSE, "code"=0, "source"=""} ("error IO"), s=w248, f=w246) -> (s? t:f=w265:errorcluster)
        n117 = global read "MH_LibVersion_global.vi" "Library Version"() -> (w244:string)
        n118 = Build Array (concatenate)(w285, w284) -> (w283:T10[])
        n119 = call "InitMH_UIThread.vi"("error in (no error)"=w265, "Mode"=w243, "refsource"=w245, "Library Version"=w244) -> ("error out"=w288:errorcluster, "Init Info"=w291:T9, "DevIdx"=w290:i32)  [unwired: 5 in]
        n120 = local write "SyncDivider"(w282) -> ()
        n121 = local write "SyncOffset"(w281) -> ()
        n122 = local write "SyncEdge"(w280) -> ()
        n123 = local write "SyncLevel"(w279) -> ()
        n124 = local write "Binning"(w278) -> ()
        n125 = local write "HistoOffset"(w277) -> ()
        n126 = Bundle By Name(cluster=w269, "DevIdx"=w290, "Init Info"=w291, "Status"="Initialized!") -> (w268:T8)
        n127 = Unbundle By Name(w268) -> ("Init Info.Bin Steps"=w267:i32, "Init Info.nchannels"=w255:i32)
        n128 = for {
          N: w255 -> [_]
          tunnel: T2 {"Name"="", "Enable"=FALSE, "Offset"=0, "Level"=10, "Edge"=50} ("Channel") -> [w303]
          tunnel: [w302] -> w287 mode=indexing
          tunnel: [w292] -> w286 mode=indexing
          i -> [w292]
          # "Init values for Inp. Channels"
          n129 = Increment(x=w292) -> (x+1=w295:i32)
          n130 = Format Into String(format string="Inp.Chan %d", w295) -> (resulting string=w300:string)  [unwired: 2 in, 1 out]
          n131 = Format Into String(format string="Ch.%d", w295) -> (resulting string=w293:string)  [unwired: 2 in, 1 out]
          n132 = property on="HistoGraph" class="WFGraph (strict)"("Active Plot"=w292, "Plot.Plot Name"=w293) -> ()  [unwired: 2 in, 2 out]
          n133 = property on="TTraceGraph" class="WFGraph (strict)"("Active Plot"=w292, "Plot.Plot Name"=w293) -> ()  [unwired: 2 in, 2 out]
          n134 = Bundle By Name(cluster=w303, "Name"=w300, "Enable"=TRUE, "Offset"=0, "Level"=-50 ("CFDZeroX"), "Edge"=0 ("CFDLevel")) -> (w302:T2)
        }
        n135 = Bundle By Name(cluster=T5 {"Histos"=[], "Cmd"=enum."_none_", "TimeTrace"=[], "Bin"=0, "Total bin"=0, "Status"="", "Resol"=0.0, "DeltaT"=0.0, "nChannels"=0} ("MH_GUIThread_QData"), "Cmd"=MH_VisThread_QCmds."nChannels", "nChannels"=w255) -> (w257:T5)
        n136 = call "MH_CalcBinningValues.vi"("Bin Steps"=w267) -> ("BinningValues"=w272:cluster{"String":string, "Value":i32}[])  [unwired: 10 in]
        n137 = property on="Binning" class="Ring (strict)"("StringsAndValues[]"=w272) -> ()  [unwired: 2 in, 2 out]
        n138 = Bundle By Name(cluster=T7 {"Cmd"=enum."Proc", "nActual"=0, "Buffer"=[], "TickCount"=0, "Param"=0} ("MH_DataProcThread_QData"), "Param"=w255, "Cmd"=MH_DataProcThread_QCmds."SetNumChannels") -> (w261:T7)
        n139 = Enqueue Element(queue=w254, element=w257) -> ()  [unwired: 2 in, 3 out]
        n140 = Enqueue Element(queue=w262, element=w261) -> ()  [unwired: 2 in, 3 out]
        n141 = local write "Channels"(w287) -> ()
        n142 = Bundle By Name(cluster=w268, "Channels"=w287, "CurrentChannels"=w286, "SyncDivider"=w282, "SyncOffset"=w281, "SyncEdge"=w280, "SyncLevel"=w279, "Binning"=w278, "HistoOffset"=w277, "AcqTime"=w276, "StopOvl."=w275, "OvlLevel"=w274, "StartMeas"=w273, "Run cont."=w271, "BitShift"=w253, "HistoAcqTime"=w252) -> (w264:T8)
        n143 = local write "AcqTime"(w276) -> ()
        n144 = local write "StopOvl."(w275) -> ()
        n145 = local write "OvlLevel"(w274) -> ()
        n146 = local write "Start"(w273) -> ()
        n147 = local write "Run continuously"(w271) -> ()
        n148 = local write "BitShift"(w253) -> ()
        n149 = local write "HistoAcqTime"(w252) -> ()
        n150 = property on="Settings" class="Bool (strict)"("Val(Sgnl)"=TRUE ("Value (Signaling)")) -> ()  [unwired: 2 in, 2 out]
        n151 = property on="Scale" class="Bool (strict)"("Val(Sgnl)"=FALSE ("Value (Signaling)")) -> ()  [unwired: 2 in, 2 out]
      }
      frame "SetInpChanEnable" {
        n152 = Unbundle By Name(w310) -> ("DevIdx"=w309:i32, "Channels"=w304:T2[], "CurrentChannels"=w305:i32[])
        n153 = for {
          tunnel: w309 -> [w317]
          shift-right: [w316] -> w308
          shift-left: errorcluster {"status"=FALSE, "code"=0, "source"=""} ("error out") -> [w315]
          tunnel: w305 -> [w311] mode=indexing
          tunnel: w304 -> [w314]
          n154 = Index Array(array=w314, index=w311) -> (element=w313:T2)
          n155 = Unbundle By Name(w313) -> ("Enable"=w312:bool)
          n156 = call "MH_SetInputChannelEnable.vi"("error in (no error)"=w315, "enable"=w312, "channel"=w311, "devidx"=w317) -> ("error out"=w316:errorcluster)  [unwired: 6 in, 1 out]
        }
      }
      frame "SetInpChanOffset" {
        n157 = Unbundle By Name(w324) -> ("DevIdx"=w323:i32, "Channels"=w318:T2[], "CurrentChannels"=w319:i32[])
        n158 = for {
          tunnel: w323 -> [w329]
          shift-right: [w326] -> w322
          shift-left: errorcluster {"status"=FALSE, "code"=0, "source"=""} ("error out") -> [w327]
          tunnel: w319 -> [w328] mode=indexing
          tunnel: w318 -> [w331]
          n159 = Index Array(array=w331, index=w328) -> (element=w330:T2)
          n160 = Unbundle By Name(w330) -> ("Offset"=w325:i32)
          n161 = call "MH_SetInputChannelOffset.vi"("error in (no error)"=w327, "Offset"=w325, "channel"=w328, "devidx"=w329) -> ("error out"=w326:errorcluster)  [unwired: 6 in, 1 out]
        }
      }
      frame "SetInpChanTrg" {
        n162 = Unbundle By Name(w338) -> ("DevIdx"=w337:i32, "Channels"=w332:T2[], "CurrentChannels"=w333:i32[])
        n163 = for {
          tunnel: w337 -> [w341]
          shift-right: [w343] -> w336
          shift-left: errorcluster {"status"=FALSE, "code"=0, "source"=""} ("error out") -> [w344]
          tunnel: w333 -> [w342] mode=indexing
          tunnel: w332 -> [w346]
          n164 = Index Array(array=w346, index=w342) -> (element=w345:T2)
          n165 = Unbundle By Name(w345) -> ("Level"=w340:i32, "Edge"=w339:i32)
          n166 = call "MH_SetInputEdgeTrg.vi"("channel"=w342, "error in (no error)"=w344, "edge"=w339, "level"=w340, "devidx"=w341) -> ("error out"=w343:errorcluster)  [unwired: 5 in, 1 out]
        }
      }
      frame "SetSyncDivider" {
        n167 = Unbundle By Name(w354) -> ("DevIdx"=w353:i32, "SyncDivider"=w349:i32)
        n168 = Power Of 2(x=w349) -> (2^x=w348:dbl)
        n169 = To Long Integer(number=w348) -> (32bit integer=w347:i32)
        n170 = call "MH_SetSyncDiv.vi"("SyncDivider"=w347, "devidx"=w353) -> ("error out"=w351:errorcluster)  [unwired: 8 in, 1 out]
        n171 = flat-sequence {
          tunnel: w351 -> [w355]
          tunnel: [w355] -> w350
          frame #0 {
            n172 = Wait (ms)(milliseconds to wait=u32 100) -> ()  [unwired: 1 out]
          }
        }
      }
      frame "SetSyncTrg" {
        n173 = Unbundle By Name(w362) -> ("DevIdx"=w359:i32, "SyncLevel"=w357:i32, "SyncEdge"=w358:i32)
        n174 = call "MH_SetSyncEdgeTrg.vi"("edge"=w358, "level"=w357, "devidx"=w359) -> ("error out"=w360:errorcluster)  [unwired: 7 in, 1 out]
      }
      frame "SetSyncOffset" {
        n175 = Unbundle By Name(w367) -> ("DevIdx"=w365:i32, "SyncOffset"=w364:i32)
        n176 = call "MH_SetSyncChannelOffset.vi"("Offset"=w364, "devidx"=w365) -> ("error out"=w366:errorcluster)  [unwired: 8 in, 1 out]
      }
      frame "SetBinning" {
        # "When binning is changed the new resolution is querried"
        n177 = Unbundle By Name(w374) -> ("DevIdx"=w372:i32, "Binning"=w371:i32)
        n178 = call "MH_SetBinning.vi"("Binning"=w371, "devidx"=w372) -> ("error out"=w373:errorcluster)  [unwired: 8 in, 1 out]
        n179 = Build Array (concatenate)(MH_UIThread_Cmds."GetResolution", w369) -> (w370:T10[])
      }
      frame "SetHistoOffset" {
        n180 = Unbundle By Name(w379) -> ("DevIdx"=w376:i32, "HistoOffset"=w375:i32)
        n181 = call "MH_SetOffset.vi"("Offset"=w375, "devidx"=w376) -> ("error out"=w377:errorcluster)  [unwired: 8 in, 1 out]
      }
      frame "SetStopOvl" {
        n182 = Unbundle By Name(w386) -> ("DevIdx"=w383:i32, "StopOvl."=w382:bool, "OvlLevel"=w381:u32)
        n183 = To Unsigned Long Integer(number=w381) -> (unsigned 32bit integer=w380:u32)
        n184 = call "MH_SetStopOverflow.vi"("stopcount"=w380, "StopOnOverflow"=w382, "devidx"=w383) -> ("error out"=w384:errorcluster)  [unwired: 7 in, 1 out]
      }
      frame "SetBitShift" {
        n185 = Unbundle By Name(w390) -> ("BitShift"=w388:i32, "SyncRate"=w389:i32)
        n186 = Negate(x=w388) -> (-x=w398:i32)
        n187 = Bundle By Name(cluster=T7 {"Cmd"=enum."Proc", "nActual"=0, "Buffer"=[], "TickCount"=0, "Param"=0} ("MH_DataProcThread_QData"), "Param"=w398, "Cmd"=MH_DataProcThread_QCmds."SetShift") -> (w404:T7)
        n188 = To Double Precision Float(number=w388) -> (double precision float=w403:dbl)
        n189 = To Double Precision Float(number=w389) -> (double precision float=w402:dbl)
        n190 = Power Of 2(x=w403) -> (2^x=w401:dbl)
        n191 = Enqueue Element(queue=w391, element=w404) -> ()  [unwired: 2 in, 3 out]
        n192 = Multiply(x=w401, y=1000.0) -> (x*y=w400:dbl)
        n193 = Divide(x=w400, y=w402) -> (x/y=w387:dbl)
        "DeltaT" <- w387
        n194 = Bundle By Name(cluster=T5 {"Histos"=[], "Cmd"=enum."_none_", "TimeTrace"=[], "Bin"=0, "Total bin"=0, "Status"="", "Resol"=0.0, "DeltaT"=0.0, "nChannels"=0} ("MH_GUIThread_QData"), "DeltaT"=w387, "Cmd"=MH_VisThread_QCmds."DeltaT") -> (w399:T5)
        n195 = Enqueue Element(queue=w392, element=w399) -> ()  [unwired: 2 in, 3 out]
      }
      frame "SetHistoAcqTime" {
        n196 = Unbundle By Name(w407) -> ("SyncRate"=w413:i32, "HistoAcqTime"=w406:dbl)
        n197 = To Double Precision Float(number=w413) -> (double precision float=w416:dbl)
        n198 = Multiply(x=w416, y=w406) -> (x*y=w415:dbl)
        n199 = Round To Nearest(number=w415) -> (nearest integer value=w414:dbl)
        n200 = To Long Integer(number=w414) -> (32bit integer=w412:i32)
        n201 = Bundle By Name(cluster=T7 {"Cmd"=enum."Proc", "nActual"=0, "Buffer"=[], "TickCount"=0, "Param"=0} ("MH_DataProcThread_QData"), "Param"=w412, "Cmd"=MH_DataProcThread_QCmds."SetHistAcqTime") -> (w411:T7)
        n202 = Enqueue Element(queue=w408, element=w411) -> ()  [unwired: 2 in, 3 out]
      }
      frame "GetAllRates" {
        # "An alternative to GetRates"
        n203 = Unbundle By Name(w421) -> ("DevIdx"=w423:i32, "Init Info.nchannels"=w426:i32)
        n204 = call "MH_AllocateCntRateBuffer.vi"("NumChan"=w426) -> ("Buffer"=w425:i32[])  [unwired: 10 in]
        n205 = call "MH_GetAllCountRates.vi"("cntrates_buf"=w425, "devidx"=w423) -> ("error out"=w420:errorcluster, "cntrates"=→"CountRates":i32[], "syncrate"=w424:i32)  [unwired: 6 in, 1 out]
        n206 = Format Into String(format string="Sync Rate: %d cps\n", w424) -> (resulting string=→"SyncRate":string)  [unwired: 2 in, 1 out]
      }
      frame "GetRates" {
        # "An alternative to GetAllRates"
        n207 = Unbundle By Name(w432) -> ("Init Info.nchannels"=w437:i32, "Channels"=w433:T2[], "DevIdx"=w434:i32)
        n208 = call "MH_GetSyncRate.vi"("devidx"=w434) -> ("error out"=w436:errorcluster, "syncrate"=w430:i32)  [unwired: 8 in, 1 out]
        n209 = Format Into String(format string="Sync Rate: %d cps\n", w430) -> (resulting string=w429:string)  [unwired: 2 in, 1 out]
        n210 = local write "SyncRate"(w429) -> ()
        n211 = for {
          N: w437 -> [_]
          tunnel: w434 -> [w445]
          tunnel: [w442] -> w428 mode=indexing
          shift-right: [w444] -> w438
          shift-left: w436 -> [w446]
          tunnel: w433 -> [w441] mode=indexing
          i -> [w443]
          n212 = Unbundle By Name(w441) -> ("Enable"=w440:bool)
          n213 = case shown="True" w440 {
            tunnel: w446 -> [w447 w452]
            tunnel: w445 -> [_ w451]
            tunnel: [w447 w450] -> w444
            tunnel: w443 -> [_ w449]
            tunnel: [_ w448] -> w442
            frame False {
            }
            frame True {
              n214 = call "MH_GetCountRate.vi"("error in (no error)"=w452, "Channel"=w449, "devidx"=w451) -> ("error out"=w450:errorcluster, "rate"=w448:i32)  [unwired: 6 in, 1 out]
            }
          }
        }
        n215 = local write "CountRates"(w428) -> ()
        n216 = Bundle By Name(cluster=w432, "SyncRate"=w430) -> (w431:T8)
      }
      frame "StartMeas" {
        n217 = Bundle By Name(cluster=T7 {"Cmd"=enum."Proc", "nActual"=0, "Buffer"=[], "TickCount"=0, "Param"=0} ("MH_DataProcThread_QData"), "Cmd"=MH_DataProcThread_QCmds."Init") -> (w454:T7)
        n218 = Unbundle By Name(w463) -> ("DevIdx"=w461:i32, "AcqTime"=w457:i32)
        n219 = Enqueue Element(queue=w456, element=w454) -> ()  [unwired: 2 in, 3 out]
        n220 = call "MH_StartMeas.vi"("tacq"=w457, "devidx"=w461) -> ("error out"=w462:errorcluster)  [unwired: 8 in, 1 out]
        n221 = Build Array (concatenate)(w460, MH_UIThread_Cmds."ReadFiFo") -> (w459:T10[])
      }
      frame "StopMeas" {
        n222 = Unbundle By Name(w469) -> ("Run cont."=w464:bool, "DevIdx"=w470:i32)
        n223 = call "MH_StopMeas.vi"("devidx"=w470) -> ("error out"=w471:errorcluster)  [unwired: 9 in, 1 out]
        n224 = case shown="True" w464 {
          tunnel: w469 -> [w475 w477]
          tunnel: [w474 w477] -> w468
          tunnel: [w472 w476] -> w467
          frame False {
            w472 = T10[] [enum."ReadFiFo"] items=["Idle", "Init", "SetInpChanEnable", "SetInpChanOffset", "SetInpChanTrg", "SetSyncDivider", "SetSyncTrg", "SetSyncOffset", "SetBinning", "SetHistoOffset", "SetHistoLen", "SetStopOvl", "SetBitShift", "SetHistoAcqTime", "GetRates", "GetAllRates", "StartMeas", "StopMeas", "AbortMeas", "GetResolution", "GetHistos", "GetAllHistos", "ReadFiFo", "WriteStatus", "Resize", "EnableControls", "DisableControls", "Error", "Exit"]
            w473 = FALSE ("StartMeas")
            n225 = Bundle By Name(cluster=w475, "StartMeas"=w473) -> (w474:T8)
            n226 = local write "Start"(w473) -> ()
          }
          frame True {
            w476 = T10[] [enum."ReadFiFo", enum."StartMeas"] items=["Idle", "Init", "SetInpChanEnable", "SetInpChanOffset", "SetInpChanTrg", "SetSyncDivider", "SetSyncTrg", "SetSyncOffset", "SetBinning", "SetHistoOffset", "SetHistoLen", "SetStopOvl", "SetBitShift", "SetHistoAcqTime", "GetRates", "GetAllRates", "StartMeas", "StopMeas", "AbortMeas", "GetResolution", "GetHistos", "GetAllHistos", "ReadFiFo", "WriteStatus", "Resize", "EnableControls", "DisableControls", "Error", "Exit"]
          }
        }
        n227 = Build Array (concatenate)(w466, w467) -> (w465:T10[])
      }
      frame "AbortMeas" {
        w479 = FALSE ("StartMeas")
        n228 = Unbundle By Name(w481) -> ("DevIdx"=w482:i32)
        n229 = call "MH_StopMeas.vi"("devidx"=w482) -> ("error out"=w483:errorcluster)  [unwired: 9 in, 1 out]
        n230 = Bundle By Name(cluster=w481, "StartMeas"=w479) -> (w480:T8)
        n231 = local write "Start"(w479) -> ()
      }
      frame "GetResolution" {
        # "Resolution in ns"
        # "Gets resolution in ps"
        # "Resolution is saved in UIThread Data cluster in ns"
        n232 = Unbundle By Name(w492) -> ("DevIdx"=w494:i32)
        n233 = call "MH_GetResolution.vi"("devidx"=w494) -> ("error out"=w493:errorcluster, "resolution"=w490:dbl)  [unwired: 8 in, 1 out]
        n234 = Divide(x=w490, y=1000.0) -> (x/y=w486:dbl)
        n235 = Bundle By Name(cluster=w492, "Resolution"=w486) -> (w491:T8)
        n236 = Bundle By Name(cluster=T5 {"Histos"=[], "Cmd"=enum."_none_", "TimeTrace"=[], "Bin"=0, "Total bin"=0, "Status"="", "Resol"=0.0, "DeltaT"=0.0, "nChannels"=0} ("MH_GUIThread_QData"), "Resol"=w486, "Cmd"=MH_VisThread_QCmds."Resol") -> (w484:T5)
        n237 = Enqueue Element(queue=w488, element=w484) -> ()  [unwired: 2 in, 3 out]
      }
      frame "ReadFiFo" {
        w504 = 2  # FLAG_FIFOFULL
        # "Reads photon records from HW and transferes them to DataProcThread via Queue."
        n238 = Unbundle By Name(w506) -> ("DevIdx"=w500:i32)
        n239 = call "MH_GetFlags.vi"("devidx"=w500) -> ("error out"=w502:errorcluster, "flags"=w503:i32)  [unwired: 8 in, 1 out]
        n240 = And(x=w503, y=w504) -> (x .and. y?=w505:i32)
        n241 = Not Equal To 0?(x=w505) -> (x != 0?=w499:bool)
        "OverRun" <- w499
        n242 = case shown="False" w499 {
          tunnel: w502 -> [w516 w519]
          tunnel: [w515 w519] -> w501
          tunnel: w500 -> [w508 _]
          tunnel: w498 -> [w514 _]
          tunnel: w497 -> [w513 _]
          tunnel: [w513 w517] -> w496
          frame False {
            n243 = call "MH_ReadFiFo.vi"("error in (no error)"=w516, "devidx"=w508) -> ("error out"=w515:errorcluster, "nactual"=w507:i32, "buffer"=w511:u32[])  [unwired: 6 in, 1 out]
            n244 = Bundle By Name(cluster=T7 {"Cmd"=enum."Proc", "nActual"=0, "Buffer"=[], "TickCount"=0, "Param"=0} ("MH_DataProcThread_QData"), "Buffer"=w511, "nActual"=w507, "Cmd"=MH_DataProcThread_QCmds."Proc") -> (w509:T7)
            n245 = Enqueue Element(queue=w514, element=w509) -> ()  [unwired: 2 in, 3 out]
          }
          frame True {
            n246 = Build Array(MH_UIThread_Cmds."AbortMeas") -> (w517:T10[])
          }
        }
      }
      frame "WriteStatus" {
        n247 = Unbundle By Name(w521) -> ("Status"=→"Status":string)
      }
      frame "Resize" {
        n248 = property on="Pane 3" class="Pane"() -> ("Width"=w528:u32)  [unwired: 2 in, 2 out]
        n249 = Subtract(x=w528, y=i16 100 ("b")) -> (x-y=w534:u32)
        n250 = Unbundle By Name(w523) -> ("Init Info.nchannels"=w531:i32)
        n251 = Quotient & Remainder(x=w534, y=i16 99 ("m")) -> (floor(x/y)=w533:u32)  [unwired: 1 out]
        n252 = In Range and Coerce(upper limit=w531, x=w533, lower limit=4) -> (coerced(x)=w532:u32)  [unwired: 1 out]
        n253 = Equal?(x=w531, y=w532) -> (x = y?=w530:bool)
        n254 = Not(x=w530) -> (.not. x?=w529:bool)
        n255 = property on="Channels" class="Arr (strict)"("HorizScroll"=w529, "Number of Columns"=w532, "Index Values"=u32[] [0]) -> ()  [unwired: 2 in, 2 out]
      }
      frame "EnableControls" {
        n256 = property class="VI"() -> ("Panel"=w539:refnum<vi>)  [unwired: 2 in, 2 out]
        n257 = property class="Pnl"(reference=w539) -> ("Controls[]"=w538:refnum<vi>[])  [unwired: 1 in, 2 out]
        n258 = property class="Pnl"(reference=w539) -> ("Decos[]"=w540:refnum<vi>[])  [unwired: 1 in, 2 out]
        n259 = for {
          tunnel: w540 -> [w544] mode=indexing
          tunnel: TRUE -> [w543]
          n260 = property class="Decor"(reference=w544, "Visible"=w543) -> ()  [unwired: 1 in, 2 out]
        }
        n261 = for {
          tunnel: w538 -> [w547] mode=indexing
          tunnel: T11."Enabled" ("Disabled") -> [w546]
          tunnel: [w545] -> _
          n262 = property class="Ctl"(reference=w547, "DisabledEnum"=w546) -> (error out=w545:errorcluster)  [unwired: 1 in, 1 out]
        }
      }
      frame "DisableControls" {
        n263 = property class="VI"() -> ("Panel"=w551:refnum<vi>)  [unwired: 2 in, 2 out]
        n264 = property class="Pnl"(reference=w551) -> ("Controls[]"=w550:refnum<vi>[])  [unwired: 1 in, 2 out]
        n265 = property class="Pnl"(reference=w551) -> ("Decos[]"=w552:refnum<vi>[])  [unwired: 1 in, 2 out]
        n266 = for {
          tunnel: w552 -> [w556] mode=indexing
          tunnel: FALSE -> [w555]
          n267 = property class="Decor"(reference=w556, "Visible"=w555) -> ()  [unwired: 1 in, 2 out]
        }
        n268 = for {
          tunnel: w550 -> [w559] mode=indexing
          tunnel: T11."Disabled and Grayed Out" ("Disabled") -> [w558]
          tunnel: [w557] -> _
          n269 = property class="Ctl"(reference=w559, "DisabledEnum"=w558) -> (error out=w557:errorcluster)  [unwired: 1 in, 1 out]
        }
      }
      frame "Error" {
        w560 = T10[] [enum."Exit"] items=["Idle", "Init", "SetInpChanEnable", "SetInpChanOffset", "SetInpChanTrg", "SetSyncDivider", "SetSyncTrg", "SetSyncOffset", "SetBinning", "SetHistoOffset", "SetHistoLen", "SetStopOvl", "SetBitShift", "SetHistoAcqTime", "GetRates", "GetAllRates", "StartMeas", "StopMeas", "AbortMeas", "GetResolution", "GetHistos", "GetAllHistos", "ReadFiFo", "WriteStatus", "Resize", "EnableControls", "DisableControls", "Error", "Exit"]
        w563 = T14 1 items=["no dialog", "OK message", "continue or stop message", "OK message + warnings", "continue/stop + warnings"] ("type of dialog (OK msg:1)")
        # "Error case: If an error occures the user is informed and the programm terminates. Add your own code to handle error events (e.g. exception lists, etc.)"
        n270 = call <vilib>:"Simple Error Handler.vi"("type of dialog (OK msg:1)"=w563, "error in (no error)"=w562) -> ()  [unwired: 3 in, 5 out]
      }
      frame "Exit" {
        n271 = Release Queue(queue=w565) -> ()  [unwired: 2 in, 3 out]
        n272 = Release Queue(queue=w564) -> ()  [unwired: 2 in, 3 out]
        n273 = Unbundle By Name(w569) -> ("DevIdx"=w568:i32)
        n274 = call "MH_CloseDevice.vi"("devidx"=w568) -> ("error out"=w567:errorcluster)  [unwired: 9 in, 1 out]
      }
    }
    n275 = call "MH_EnQError.vi"("error in (no error)"=w24, "Cmds_in"=w22) -> ("error out"=w23:errorcluster, "Cmds_out"=w21:T10[])  [unwired: 8 in]
  }
  n276 = call "MH_DataProcThread.vi"("MH_VisThread_QRef"=w7, "MH_DataProcThread_QRef"=w1) -> ()  [unwired: 10 in]
  n277 = while {
    tunnel: w7 -> [w578]
    shift-right: [w574] -> _
    shift-left: T4 {"Resol"=0.0, "DeltaT"=0.0, "NumChannels"=0} -> [w575]
    tunnel: w1 -> [w573]
    stop <- w571 stop-if-true
    # "VisualizationThread"
    n278 = Dequeue Element(queue=w578, timeout in ms (-1)=100) -> (element=w576:T5, error out=w571:errorcluster)  [unwired: 1 in, 2 out]
    n279 = Unbundle By Name(w576) -> ("Cmd"=w577:T6)
    n280 = case shown="\"Histo\"" w577 {
      tunnel: w576 -> [_ w591 w593 w605 w613 w617 w621]
      tunnel: w575 -> [w581 w589 w595 w597 w612 w616 w620]
      tunnel: [w581 w589 w594 w597 w612 w615 w619] -> w574
      tunnel: w573 -> [w580 _ _ _ w609 _ _]
      tunnel: w571 -> [w579 _ _ _ _ _ _]
      frame "_none_", Default {
        n281 = case shown="No Error" w579 {
          tunnel: w580 -> [w585 _]
          frame No Error {
            n282 = Get Queue Status(queue=w585) -> (# elements in queue=w583:i32)  [unwired: 2 in, 7 out]
            n283 = Format Into String(format string="Elements in Q: %d", w583) -> (resulting string=w582:string)  [unwired: 2 in, 1 out]
            n284 = local write "Status"(w582) -> ()
          }
          frame Error {
          }
        }
      }
      frame "Histo" {
        n285 = Unbundle By Name(w591) -> ("Histos"=w586:u32[][])
        n286 = Unbundle By Name(w589) -> ("Resol"=w588:dbl)
        n287 = Bundle(0.0, "Resol"=w588, "Histos"=w586) -> (→"HistoGraph":cluster{dbl, "Resol":dbl, "Histos":u32[][]})  [unwired: 1 in]
      }
      frame "nChannels" {
        n288 = Unbundle By Name(w593) -> ("nChannels"=w592:i32)
        n289 = Bundle By Name(cluster=w595, "NumChannels"=w592) -> (w594:T4)
      }
      frame "TTrace" {
        n290 = Unbundle By Name(w605) -> ("Total bin"=w604:u64, "Bin"=w603:i32, "TimeTrace"=w602:u32[][])
        n291 = Unbundle By Name(w597) -> ("DeltaT"=w596:dbl)
        n292 = call "MH_TTraceToGraph.vi"("DeltaT"=w596, "TimeTrace"=w602, "Bin"=w603, "Total bin"=w604) -> ("TimeTrace_out"=w599:u32[][], "dt"=w600:dbl, "T0"=w601:dbl)  [unwired: 5 in]
        n293 = Bundle("T0"=w601, "dt"=w600, "TimeTrace_out"=w599) -> (→"TTraceGraph":T15)  [unwired: 1 in]
      }
      frame "Status" {
        n294 = Unbundle By Name(w613) -> ("Status"=w610:string)
        n295 = Get Queue Status(queue=w609) -> (# elements in queue=w608:i32)  [unwired: 2 in, 7 out]
        n296 = Format Into String(format string="\t\tElements in Q: %d", w608) -> (resulting string=w606:string)  [unwired: 2 in, 1 out]
        n297 = Concatenate Strings(w610, w606) -> (w611:string)
        n298 = local write "Status"(w611) -> ()
      }
      frame "DeltaT" {
        n299 = Unbundle By Name(w617) -> ("DeltaT"=w614:dbl)
        n300 = Bundle By Name(cluster=w616, "DeltaT"=w614) -> (w615:T4)
      }
      frame "Resol" {
        n301 = Unbundle By Name(w621) -> ("Resol"=w618:dbl)
        n302 = Bundle By Name(cluster=w620, "Resol"=w618) -> (w619:T4)
      }
    }
  }
